vi "Convert Spectrum to DBFS.vi"(8 "error in (no error)":errorcluster, 11 "Spectral Information":dbl[](array[numeric])) -> (0 "error out":errorcluster, 3 "Spectral Information Out (DBFS)":dbl[](array[numeric]))   [LabVIEW 2017]
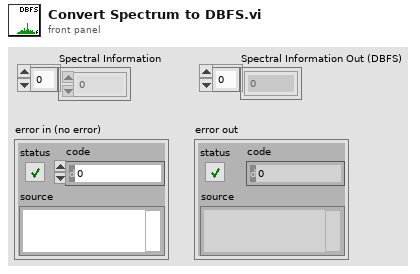
[diagram p1: front panel]
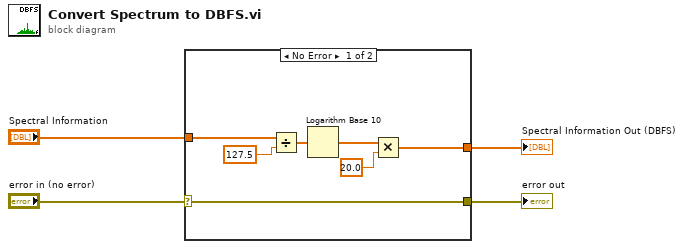
[diagram p0: block diagram]
diagram:
  n1 = case shown="No Error" "error in (no error)" {
    selector: "error in (no error)" -> [w5 w12]
    tunnel: [w9 w13] -> w4
    tunnel: "Spectral Information" -> [w6 w13]
    tunnel: [w5 w12] -> w1
    frame No Error {
      n2 = Divide(x=w6, y=127.5) -> (x/y=w11:dbl[])
      n3 = Logarithm Base 10(1:w11) -> (0:w7:dbl[])
      n4 = Multiply(x=w7, y=20.0) -> (x*y=w9:dbl[])
    }
    frame Error {
    }
  }
  "Spectral Information Out (DBFS)" <- w4
  "error out" <- w1
